vi "Swerve Check for New Command.vi"(8 "Current Command":T6, 10 "Wait time (ms)":dbl, 11 "Finished?":bool) -> (0 "Completion":T4, 1 "Subsystem Name":string, 2 "Current Command":T1, 3 "Initial Trace String":string, 4 "NextCommand":T6)   [LabVIEW 2020]
doc: "This VI is called for each controller loop iteration. It checks for new commands, updates timing data, and upon completion, notifies any waiting commands."
uses:
  Swerve Setpoints.ctl
  Swerve Operations.ctl
  <vilib>/Rock Robotics/WPI/Framework/Command Status Info.ctl
  <vilib>/Rock Robotics/WPI/Framework/Completion Status.ctl
  <vilib>/Rock Robotics/WPI/Framework/Completion Notifier.ctl
  Swerve Published Globals.vi
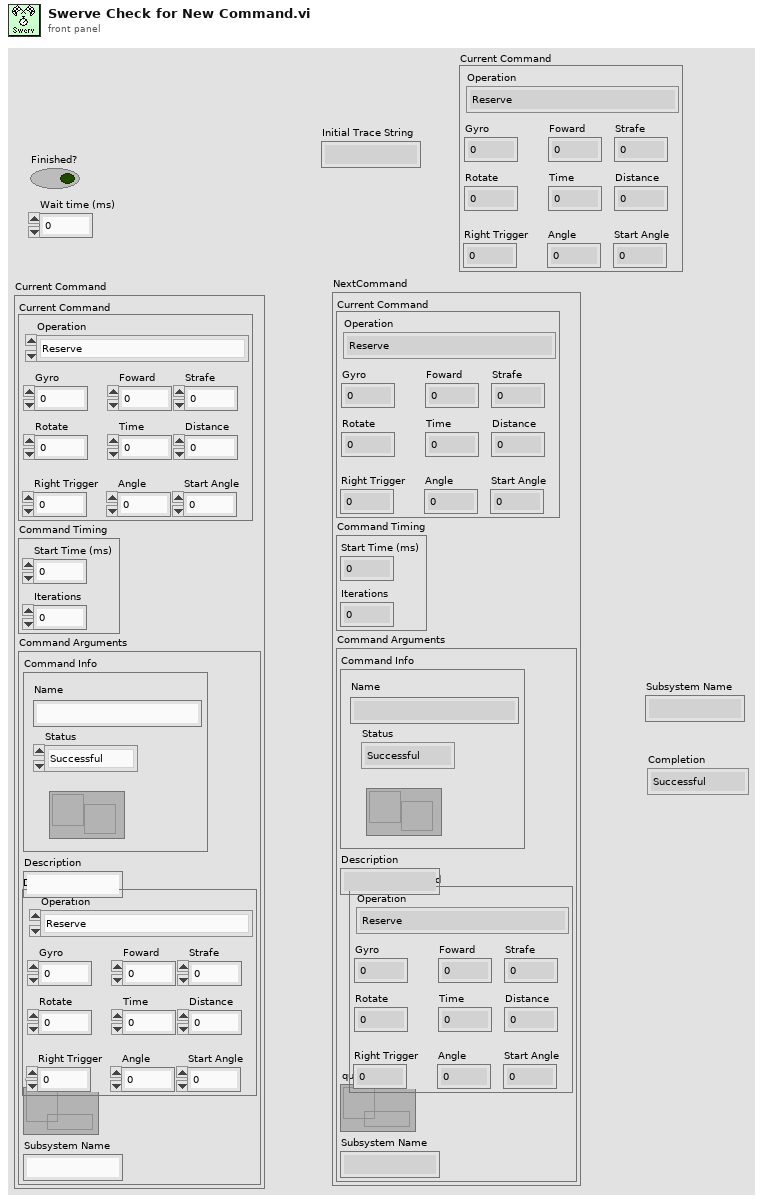
[diagram p1: front panel]
types:
  T1 = typedef "Swerve Setpoints.ctl" = cluster{"Operation":T2, "Gyro":dbl, "Rotate":dbl, "Time":dbl, "Foward":dbl, "Distance":dbl, "Strafe":dbl, "Right Trigger":dbl, "Angle":dbl, "Start Angle":dbl}
  T2 = typedef "Swerve Operations.ctl" = enum16{"Reserve", "Read Current", "Immediate", "Joystick Drive", "Drive for Time", "Turn to Angle", "Drive to Angle(Time)", "Drive for Distance", "Drive to Angle(Distance)"}
  T3 = typedef "Command Status Info.ctl" = cluster{"Name":string, "Status":T4, "notifier out":T5}
  T4 = typedef "Completion Status.ctl" = enum16{"Successful", "Aborted", "Incomplete"}
  T5 = typedef "Completion Notifier.ctl" = refnum<notifier>
  T6 = cluster{"Current Command":T1, "Command Timing":cluster{"Start Time (ms)":u32, "Iterations":i32}, "Command Arguments":cluster{"Command Info":T3, "Description":string, "Default Command":T1, "queue out":refnum<queue>, "Subsystem Name":string}}
  T7 = cluster{"Command Info":T3, "Description":string, "Default Command":T1, "queue out":refnum<queue>, "Subsystem Name":string}
  T8 = cluster{"Default Command":T1, "Command Info":T3, "Description":string}
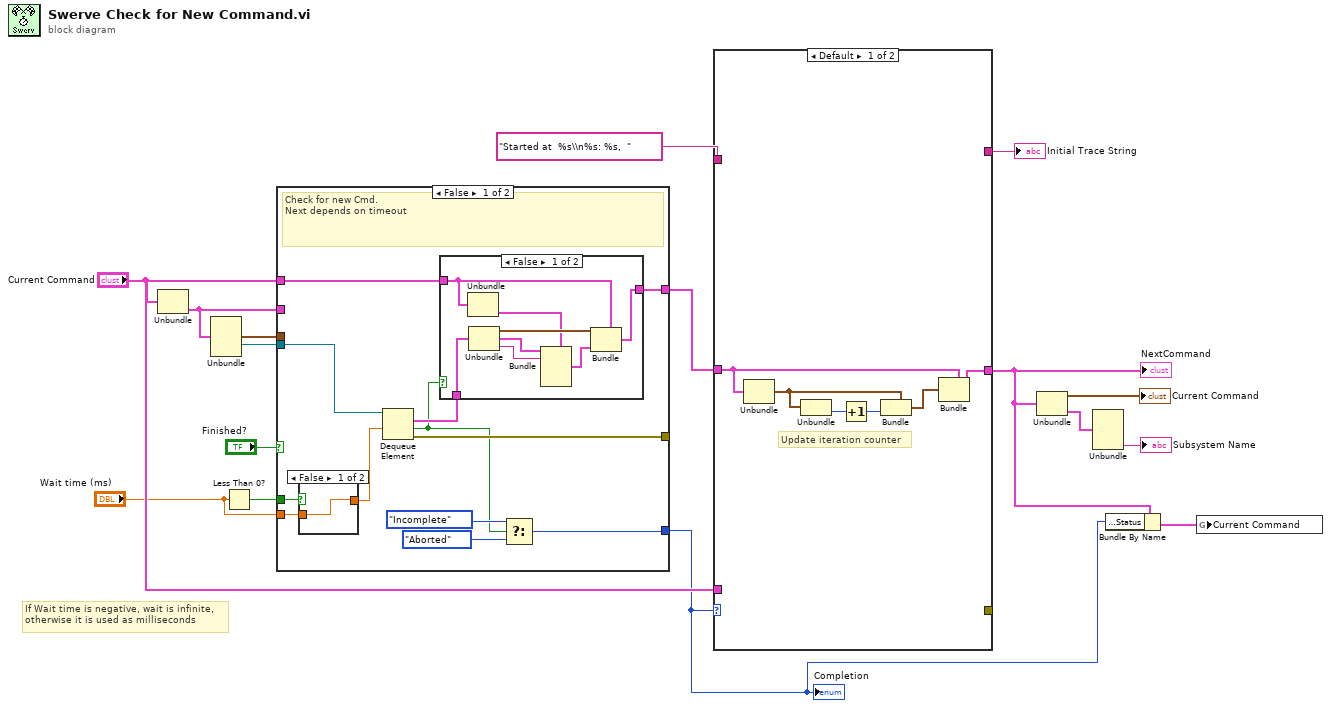
[diagram p0: block diagram]
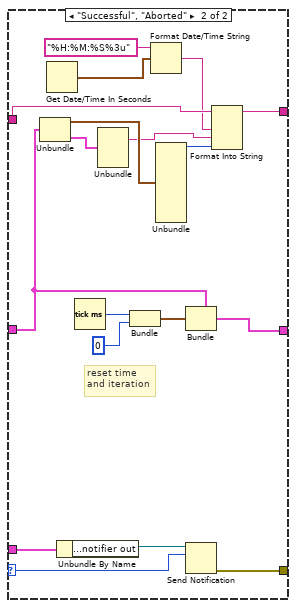
[diagram p2: hidden frame]
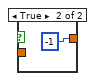
[diagram p4: hidden frame]
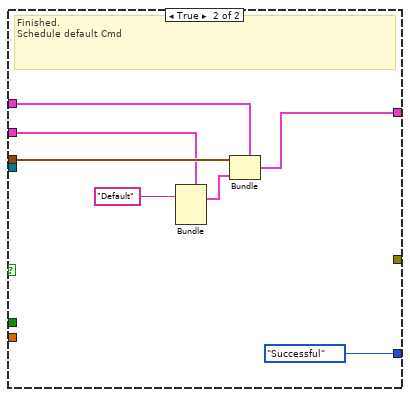
[diagram p5: hidden frame]
diagram:
  # "If Wait time is negative, wait is infinite,\notherwise it is used as milliseconds"
  n1 = Unbundle("Current Command") -> ("Command Arguments"=w6:T7)  [unwired: 2 out]
  n2 = Unbundle(w6) -> ("Default Command"=w9:T1, "queue out"=w10:refnum<queue>)  [unwired: 3 out]
  n3 = Less Than 0?(x="Wait time (ms)") -> (x < 0?=w4:bool)
  n4 = case shown="False" "Finished?" {
    tunnel: [w23 w45] -> w13
    tunnel: w4 -> [w25 _]
    tunnel: [w28 Completion_Status."Successful"] -> w1
    tunnel: [w20 _] -> _
    tunnel: w10 -> [w22 _]
    tunnel: "Current Command" -> [w24 w44]
    tunnel: w9 -> [_ w43]
    tunnel: w6 -> [_ w41]
    tunnel: "Wait time (ms)" -> [w17 _]
    frame False {
      # "Check for new Cmd.\nNext depends on timeout"
      n5 = case shown="False" w25 {
        tunnel: [w38 -1] -> w21
        tunnel: w17 -> [w38 _]
        frame False {
        }
        frame True {
        }
      }
      n6 = Dequeue Element(queue=w22, timeout in ms (-1)=w21) -> (element=w19:T8, timed out?=w18:bool, error out=w20:errorcluster)  [unwired: 1 in, 1 out]
      n7 = case shown="False" w18 {
        tunnel: w19 -> [w36 _]
        tunnel: w24 -> [w33 w37]
        tunnel: [w29 w37] -> w23
        frame False {
          n8 = Unbundle(w33) -> ("Command Arguments"=w32:T7)  [unwired: 2 out]
          n9 = Unbundle(w36) -> ("Default Command"=w35:T1, "Command Info"=w30:T3, "Description"=w31:string)
          n10 = Bundle(cluster=w32, "Command Info"=w30, "Description"=w31) -> (w34:T7)  [unwired: 3 in]
          n11 = Bundle(cluster=w33, "Current Command"=w35, "Command Arguments"=w34) -> (w29:T6)  [unwired: 1 in]
        }
        frame True {
        }
      }
      n12 = Select(t=Completion_Status."Incomplete", s=w18, f=Completion_Status."Aborted") -> (s? t:f=w28:T4)
    }
    frame True {
      # "Finished.\nSchedule default Cmd"
      n13 = Bundle(cluster=w41, "Description"="Default") -> (w42:T7)  [unwired: 4 in]
      n14 = Bundle(cluster=w44, "Current Command"=w43, "Command Arguments"=w42) -> (w45:T6)  [unwired: 1 in]
    }
  }
  "Completion" <- w1
  n15 = case shown="Default" w1 {
    selector: w1 -> [_ w70]
    tunnel: "Current Command" -> [_ w67]
    tunnel: "Started at  %s\\n%s: %s,  " ("format string") -> [_ w66]
    tunnel: [_ w65] -> w15
    tunnel: w13 -> [w49 w54]
    tunnel: [w50 w61] -> w5
    tunnel: [_ w58] -> _
    frame Default {
      # "Update iteration counter"
      n16 = Unbundle(w49) -> ("Command Timing"=w48:cluster{"Start Time (ms)":u32, "Iterations":i32})  [unwired: 2 out]
      n17 = Unbundle(w48) -> ("Iterations"=w51:i32)  [unwired: 1 out]
      n18 = Increment(x=w51) -> (x+1=w52:i32)
      n19 = Bundle(cluster=w48, "Iterations"=w52) -> (w47:cluster{"Start Time (ms)":u32, "Iterations":i32})  [unwired: 1 in]
      n20 = Bundle(cluster=w49, "Command Timing"=w47) -> (w50:T6)  [unwired: 2 in]
    }
    frame "Successful", "Aborted" {
      # "reset time\nand iteration"
      n21 = Unbundle(w54) -> ("Current Command"=w64:T1, "Command Arguments"=w59:T7)  [unwired: 1 out]
      n22 = Get Date/Time In Seconds() -> (seconds since 1Jan1904=w57:timestamp)
      n23 = Unbundle By Name(w67) -> ("Command Arguments.Command Info.notifier out"=w69:T5)
      n24 = Tick Count (ms)() -> (millisecond timer value=w63:u32)
      n25 = Unbundle(w59) -> ("Description"=w56:string)  [unwired: 4 out]
      n26 = Bundle("millisecond timer value"=w63, 0) -> (w60:cluster{"millisecond timer value":u32, i32})  [unwired: 1 in]
      n27 = Format Date/Time String(time format string (%c)="%H:%M:%S%3u", seconds (now)=w57) -> (date/time string=w55:string)  [unwired: 1 in]
      n28 = Unbundle(w64) -> ("Operation"=w68:T2)  [unwired: 9 out]
      n29 = Bundle(cluster=w54, "Command Timing"=w60) -> (w61:T6)  [unwired: 2 in]
      n30 = Send Notification(notification=w70, notifier=w69) -> (error out=w58:errorcluster)  [unwired: 1 in, 1 out]
      n31 = Format Into String(format string=w66, w55, w56, w68) -> (resulting string=w65:string)  [unwired: 2 in, 1 out]
    }
  }
  "NextCommand" <- w5
  "Initial Trace String" <- w15
  n32 = Unbundle(w5) -> ("Current Command"=→"Current Command":T1, "Command Arguments"=w8:T7)  [unwired: 1 out]
  n33 = Unbundle(w8) -> ("Subsystem Name"=→"Subsystem Name":string)  [unwired: 4 out]
  n34 = Bundle By Name(cluster=w5, "Command Arguments.Command Info.Status"=w1) -> (w2:T6)
  n35 = global write "Swerve Published Globals.vi" "Current Command"(w2) -> ()
